vi "..gait set up data vi.vi"() -> ()   [LabVIEW 2018]
uses:
  <vilib>/Analysis/baseanly.llb/Mean (DBL).vi
  <vilib>/University of Leeds/Kinesthesia Toolkit for Microsoft Kinect/_Polymorphic Configure/Event-Skeleton and Video.vi
  <vilib>/University of Leeds/Kinesthesia Toolkit for Microsoft Kinect/_Polymorphic Read/Read-Skeleton and Video.vi
  <vilib>/Utility/file.llb/Write Delimited Spreadsheet (DBL).vi
  <vilib>/University of Leeds/Kinesthesia Toolkit for Microsoft Kinect/_Polymorphic Close/Close-Skeleton and Video.vi
  <vilib>/Utility/file.llb/Read Delimited Spreadsheet (DBL).vi
  <vilib>/Analysis/NI_AALBase.lvlib
panel:
  out "mean calculated":dbl[](array[numeric])
  out "skeleton":refnum<vi>(3d-picture)
  out "?":picture
  out "real time data":dbl[](array[numeric])
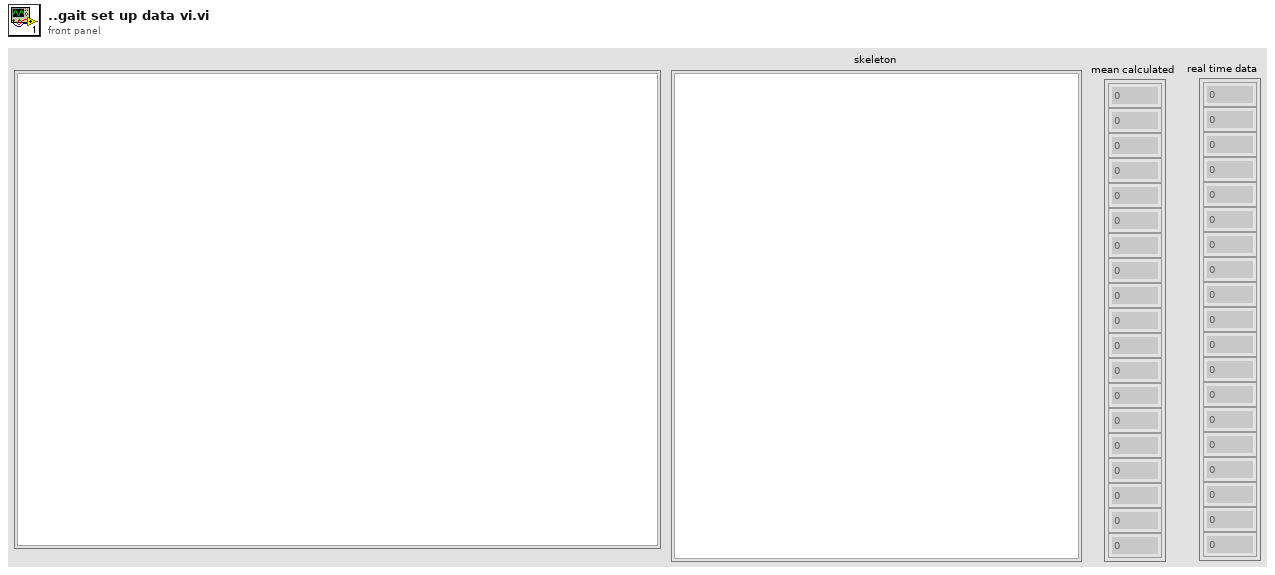
[diagram p1: front panel]
types:
  T1 = enum16{"hip centre", "spine", "shoulder centre", "head", "shoulder left", "elbow left", "wrist left", "hand left", "shoulder right", "elbow right", "wrist right", "hand right", "hip left", "knee left", "ankle left", "foot left", "hip right", "knee right", "ankle right", "foot right"}
  T2 = cluster{cluster{"reference out":refnum<k24>, "KinectSensors":refnum<k24>}, "get_Item":refnum<k24>}
  T3 = cluster{"reference out":refnum<k24>, "KinectSensors":refnum<k24>, "SkeletonStream":refnum<k24>, "ColorStream":refnum<k24>, refnum<k24>[], "get_Item":refnum<k24>}
  T4 = cluster{"Scene":refnum<vi>, "Joints":refnum<vi>[], "Bones":refnum<vi>[]}
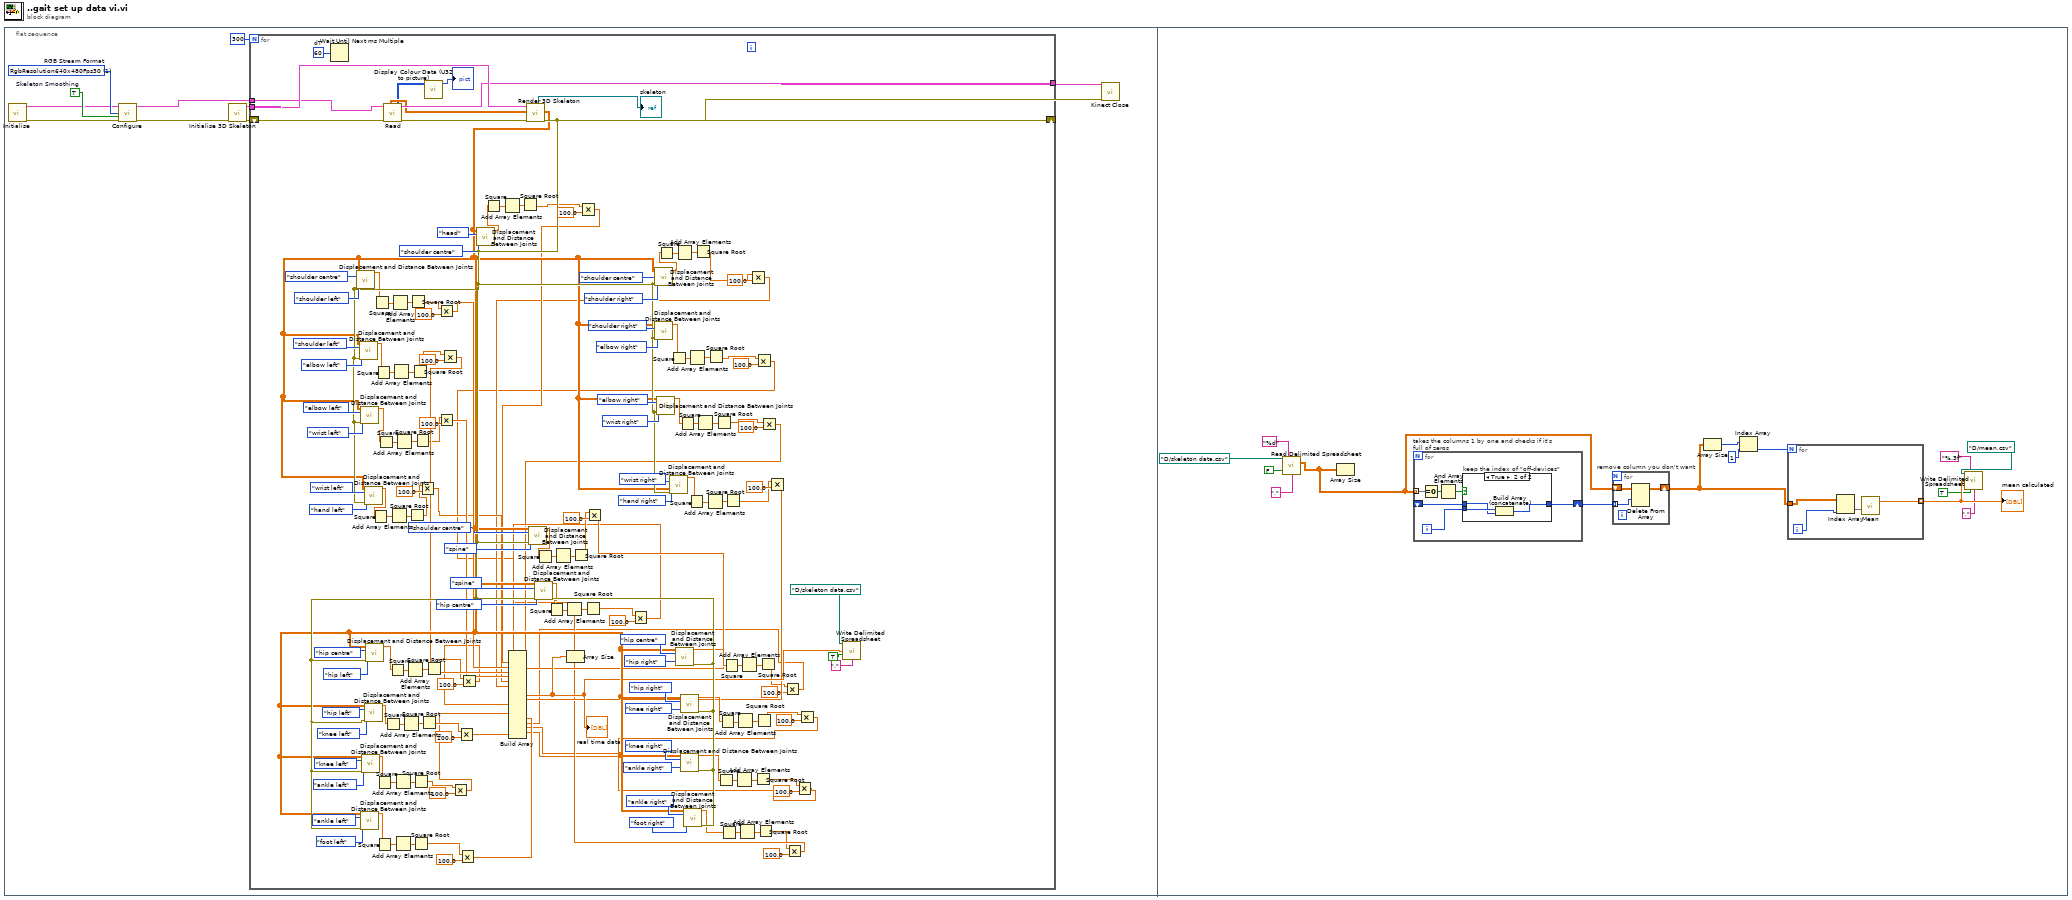
[diagram p0: block diagram]
diagram:
  n1 = flat-sequence {
    frame #0 {
      w7 = 1 items=["Undefined", "RgbResolution640x480Fps30", "RgbResolution1280x960Fps12", "YuvResolution640x480Fps15", "RawYuvResolution640x480Fps15"]  # RGB Stream Format
      w6 = TRUE  # Skeleton Smoothing
      n2 = call <vilib>:"Initialise.vi"() -> ("Kinect References out"=w2:T2, "error out"=w3:errorcluster)  [unwired: 14 in]
      n3 = call-poly <vilib>:"Configure.vi"("Kinect References in"=w2, "RGB Stream Format"=w7, "Skeleton Smoothing"=w6, "error in"=w3) -> ("Kinect References out"=w8:T3, "error out"=w9:errorcluster)  [unwired: 10 in]
      n4 = call <vilib>:"Initialise 3D Skeleton.vi"("error in (no error)"=w9) -> ("error out"=w10:errorcluster, "Scene & Skeleton Refs"=w11:T4)  [unwired: 9 in]
      n5 = for {
        N: 300 -> [_]
        tunnel: [w172] -> w4
        tunnel: w11 -> [w179]
        tunnel: w8 -> [w173]
        shift-right: [w131] -> w5
        shift-left: w10 -> [w175]
        w177 = u32 60  # dT
        n6 = Wait Until Next ms Multiple(millisecond multiple=w177) -> ()  [unwired: 1 out]
        n7 = call-poly <vilib>:"Read.vi"("Kinect References in"=w173, "error in (no error)"=w175) -> ("Primary Skeleton Array"=w171:dbl[][], "Colour output array (U24, RGB)"=w170:u32[][], "Kinect References out"=w172:T3, "error out"=w174:errorcluster)  [unwired: 9 in, 1 out]
        n8 = call <vilib>:"Display Colour Data (U32 to picture).vi"("Colour output array (U24, RGB)"=w170) -> ("new picture"=→"?":picture)  [unwired: 10 in]
        n9 = call <vilib>:"Render 3D Skeleton.vi"("error in (no error)"=w174, "Array of Joint Positions"=w171, "Scene & Skeleton Refs In"=w179) -> ("error out"=w131:errorcluster, "Array of Joint Positions Out"=w130:dbl[][], "Scene Out"=→"skeleton":refnum<vi>)  [unwired: 5 in, 1 out]
        n10 = call <vilib>:"Displacement and Distance Between Joints.vi"("Array of Joint Positions"=w130, "Joint 1"=T1."shoulder centre", "Joint 2"=T1."shoulder left", "error in (no error)"=w131) -> ("X Y Z Displacement Between Joints 1 and 2"=w121:dbl[])  [unwired: 10 in, 1 out]
        n11 = call <vilib>:"Displacement and Distance Between Joints.vi"("Array of Joint Positions"=w130, "Joint 1"=T1."shoulder left", "Joint 2"=T1."elbow left", "error in (no error)"=w131) -> ("X Y Z Displacement Between Joints 1 and 2"=w118:dbl[])  [unwired: 10 in, 1 out]
        n12 = call <vilib>:"Displacement and Distance Between Joints.vi"("Array of Joint Positions"=w130, "Joint 1"=T1."elbow left", "Joint 2"=T1."wrist left", "error in (no error)"=w131) -> ("X Y Z Displacement Between Joints 1 and 2"=w112:dbl[])  [unwired: 10 in, 1 out]
        n13 = call <vilib>:"Displacement and Distance Between Joints.vi"("Array of Joint Positions"=w130, "Joint 1"=T1."ankle left", "Joint 2"=T1."foot left", "error in (no error)"=w131) -> ("X Y Z Displacement Between Joints 1 and 2"=w85:dbl[])  [unwired: 10 in, 1 out]
        n14 = call <vilib>:"Displacement and Distance Between Joints.vi"("Array of Joint Positions"=w130, "Joint 1"=T1."knee left", "Joint 2"=T1."ankle left", "error in (no error)"=w131) -> ("X Y Z Displacement Between Joints 1 and 2"=w86:dbl[])  [unwired: 10 in, 1 out]
        n15 = call <vilib>:"Displacement and Distance Between Joints.vi"("Array of Joint Positions"=w130, "Joint 1"=T1."wrist left", "Joint 2"=T1."hand left", "error in (no error)"=w131) -> ("X Y Z Displacement Between Joints 1 and 2"=w102:dbl[])  [unwired: 10 in, 1 out]
        n16 = call <vilib>:"Displacement and Distance Between Joints.vi"("Array of Joint Positions"=w130, "Joint 1"=T1."hip left", "Joint 2"=T1."knee left", "error in (no error)"=w131) -> ("X Y Z Displacement Between Joints 1 and 2"=w87:dbl[])  [unwired: 10 in, 1 out]
        n17 = call <vilib>:"Displacement and Distance Between Joints.vi"("Array of Joint Positions"=w130, "Joint 1"=T1."hip centre", "Joint 2"=T1."hip left", "error in (no error)"=w131) -> ("X Y Z Displacement Between Joints 1 and 2"=w94:dbl[])  [unwired: 10 in, 1 out]
        n18 = Square(x=w102) -> (x^2=w106:dbl[])
        n19 = Square(x=w121) -> (x^2=w123:dbl[])
        n20 = Square(x=w118) -> (x^2=w120:dbl[])
        n21 = Square(x=w86) -> (x^2=w91:dbl[])
        n22 = Square(x=w85) -> (x^2=w89:dbl[])
        n23 = Square(x=w112) -> (x^2=w114:dbl[])
        n24 = Square(x=w87) -> (x^2=w93:dbl[])
        n25 = Square(x=w94) -> (x^2=w96:dbl[])
        n26 = Add Array Elements(numeric array=w106) -> (sum=w105:dbl)
        n27 = Add Array Elements(numeric array=w123) -> (sum=w122:dbl)
        n28 = Add Array Elements(numeric array=w120) -> (sum=w119:dbl)
        n29 = Add Array Elements(numeric array=w91) -> (sum=w90:dbl)
        n30 = Add Array Elements(numeric array=w89) -> (sum=w88:dbl)
        n31 = Add Array Elements(numeric array=w114) -> (sum=w113:dbl)
        n32 = Add Array Elements(numeric array=w93) -> (sum=w92:dbl)
        n33 = Add Array Elements(numeric array=w96) -> (sum=w95:dbl)
        n34 = Square Root(x=w105) -> (sqrt(x)=w55:dbl)
        n35 = Square Root(x=w122) -> (sqrt(x)=w63:dbl)
        n36 = Square Root(x=w119) -> (sqrt(x)=w60:dbl)
        n37 = Square Root(x=w90) -> (sqrt(x)=w28:dbl)
        n38 = Square Root(x=w88) -> (sqrt(x)=w25:dbl)
        n39 = Square Root(x=w113) -> (sqrt(x)=w57:dbl)
        n40 = Multiply(x=w55, y=100.0) -> (x*y=w54:dbl)
        n41 = Square Root(x=w92) -> (sqrt(x)=w31:dbl)
        n42 = Square Root(x=w95) -> (sqrt(x)=w34:dbl)
        n43 = Multiply(x=w63, y=100.0) -> (x*y=w64:dbl)
        n44 = Multiply(x=w57, y=100.0) -> (x*y=w58:dbl)
        n45 = Multiply(x=w60, y=100.0) -> (x*y=w61:dbl)
        n46 = Multiply(x=w28, y=100.0) -> (x*y=w27:dbl)
        n47 = Multiply(x=w31, y=100.0) -> (x*y=w30:dbl)
        n48 = Multiply(x=w25, y=100.0) -> (x*y=w24:dbl)
        n49 = Multiply(x=w34, y=100.0) -> (x*y=w33:dbl)
        n50 = call <vilib>:"Displacement and Distance Between Joints.vi"("Array of Joint Positions"=w130, "Joint 1"=T1."head", "Joint 2"=T1."shoulder centre", "error in (no error)"=w131) -> ("X Y Z Displacement Between Joints 1 and 2"=w127:dbl[])  [unwired: 10 in, 1 out]
        n51 = Square(x=w127) -> (x^2=w129:dbl[])
        n52 = Add Array Elements(numeric array=w129) -> (sum=w128:dbl)
        n53 = Square Root(x=w128) -> (sqrt(x)=w66:dbl)
        n54 = call <vilib>:"Displacement and Distance Between Joints.vi"("Array of Joint Positions"=w130, "Joint 1"=T1."shoulder centre", "Joint 2"=T1."spine", "error in (no error)"=w131) -> ("X Y Z Displacement Between Joints 1 and 2"=w100:dbl[])  [unwired: 10 in, 1 out]
        n55 = call <vilib>:"Displacement and Distance Between Joints.vi"("Array of Joint Positions"=w130, "Joint 1"=T1."spine", "Joint 2"=T1."hip centre", "error in (no error)"=w131) -> ("X Y Z Displacement Between Joints 1 and 2"=w97:dbl[])  [unwired: 10 in, 1 out]
        n56 = Square(x=w100) -> (x^2=w108:dbl[])
        n57 = Square(x=w97) -> (x^2=w99:dbl[])
        n58 = Add Array Elements(numeric array=w108) -> (sum=w107:dbl)
        n59 = Add Array Elements(numeric array=w99) -> (sum=w98:dbl)
        n60 = Square Root(x=w107) -> (sqrt(x)=w52:dbl)
        n61 = Multiply(x=w66, y=100.0) -> (x*y=w67:dbl)
        n62 = Square Root(x=w98) -> (sqrt(x)=w48:dbl)
        n63 = Multiply(x=w52, y=100.0) -> (x*y=w51:dbl)
        n64 = Multiply(x=w48, y=100.0) -> (x*y=w49:dbl)
        n65 = call <vilib>:"Displacement and Distance Between Joints.vi"("Array of Joint Positions"=w130, "Joint 1"=T1."shoulder centre", "Joint 2"=T1."shoulder right", "error in (no error)"=w131) -> ("X Y Z Displacement Between Joints 1 and 2"=w124:dbl[])  [unwired: 10 in, 1 out]
        n66 = call <vilib>:"Displacement and Distance Between Joints.vi"("Array of Joint Positions"=w130, "Joint 1"=T1."shoulder right", "Joint 2"=T1."elbow right", "error in (no error)"=w131) -> ("X Y Z Displacement Between Joints 1 and 2"=w115:dbl[])  [unwired: 10 in, 1 out]
        n67 = call <vilib>:"Displacement and Distance Between Joints.vi"("Array of Joint Positions"=w130, "Joint 1"=T1."elbow right", "Joint 2"=T1."wrist right", "error in (no error)"=w131) -> ("X Y Z Displacement Between Joints 1 and 2"=w109:dbl[])  [unwired: 10 in, 1 out]
        n68 = Square(x=w124) -> (x^2=w126:dbl[])
        n69 = call <vilib>:"Displacement and Distance Between Joints.vi"("Array of Joint Positions"=w130, "Joint 1"=T1."wrist right", "Joint 2"=T1."hand right", "error in (no error)"=w131) -> ("X Y Z Displacement Between Joints 1 and 2"=w101:dbl[])  [unwired: 10 in, 1 out]
        n70 = Square(x=w115) -> (x^2=w117:dbl[])
        n71 = Add Array Elements(numeric array=w126) -> (sum=w125:dbl)
        n72 = call <vilib>:"Displacement and Distance Between Joints.vi"("Array of Joint Positions"=w130, "Joint 1"=T1."hip centre", "Joint 2"=T1."hip right", "error in (no error)"=w131) -> ("X Y Z Displacement Between Joints 1 and 2"=w82:dbl[])  [unwired: 10 in, 1 out]
        n73 = Square(x=w109) -> (x^2=w111:dbl[])
        n74 = call <vilib>:"Displacement and Distance Between Joints.vi"("Array of Joint Positions"=w130, "Joint 1"=T1."hip right", "Joint 2"=T1."knee right", "error in (no error)"=w131) -> ("X Y Z Displacement Between Joints 1 and 2"=w75:dbl[])  [unwired: 10 in, 1 out]
        n75 = call <vilib>:"Displacement and Distance Between Joints.vi"("Array of Joint Positions"=w130, "Joint 1"=T1."knee right", "Joint 2"=T1."ankle right", "error in (no error)"=w131) -> ("X Y Z Displacement Between Joints 1 and 2"=w74:dbl[])  [unwired: 10 in, 1 out]
        n76 = call <vilib>:"Displacement and Distance Between Joints.vi"("Array of Joint Positions"=w130, "Joint 1"=T1."ankle right", "Joint 2"=T1."foot right", "error in (no error)"=w131) -> ("X Y Z Displacement Between Joints 1 and 2"=w73:dbl[])  [unwired: 10 in, 1 out]
        n77 = Square(x=w101) -> (x^2=w104:dbl[])
        n78 = Add Array Elements(numeric array=w117) -> (sum=w116:dbl)
        n79 = Square Root(x=w125) -> (sqrt(x)=w46:dbl)
        n80 = Add Array Elements(numeric array=w111) -> (sum=w110:dbl)
        n81 = Add Array Elements(numeric array=w104) -> (sum=w103:dbl)
        n82 = Square Root(x=w116) -> (sqrt(x)=w42:dbl)
        n83 = Square Root(x=w110) -> (sqrt(x)=w40:dbl)
        n84 = Square(x=w74) -> (x^2=w79:dbl[])
        n85 = Square(x=w75) -> (x^2=w81:dbl[])
        n86 = Square(x=w73) -> (x^2=w76:dbl[])
        n87 = Square(x=w82) -> (x^2=w84:dbl[])
        n88 = Square Root(x=w103) -> (sqrt(x)=w37:dbl)
        n89 = Add Array Elements(numeric array=w79) -> (sum=w78:dbl)
        n90 = Add Array Elements(numeric array=w81) -> (sum=w80:dbl)
        n91 = Add Array Elements(numeric array=w76) -> (sum=w77:dbl)
        n92 = Add Array Elements(numeric array=w84) -> (sum=w83:dbl)
        n93 = Multiply(x=w46, y=100.0) -> (x*y=w45:dbl)
        n94 = Square Root(x=w78) -> (sqrt(x)=w18:dbl)
        n95 = Multiply(x=w42, y=100.0) -> (x*y=w43:dbl)
        n96 = Square Root(x=w80) -> (sqrt(x)=w16:dbl)
        n97 = Square Root(x=w77) -> (sqrt(x)=w21:dbl)
        n98 = Square Root(x=w83) -> (sqrt(x)=w13:dbl)
        n99 = Multiply(x=w40, y=100.0) -> (x*y=w39:dbl)
        n100 = Multiply(x=w37, y=100.0) -> (x*y=w36:dbl)
        n101 = Multiply(x=w13, y=100.0) -> (x*y=w12:dbl)
        n102 = Multiply(x=w21, y=100.0) -> (x*y=w22:dbl)
        n103 = Multiply(x=w18, y=100.0) -> (x*y=w19:dbl)
        n104 = Multiply(x=w16, y=100.0) -> (x*y=w15:dbl)
        n105 = Build Array(w49, w51, w67, w64, w61, w58, w54, w45, w43, w39, w36, w33, w30, w27, w24, w12, w15, w19, w22) -> (w69:dbl[])
        "real time data" <- w69
        n106 = Array Size(array=w69) -> ()  [unwired: 1 out]
        n107 = call-poly <vilib>:"Write Delimited Spreadsheet.vi"("file path (dialog if empty)"=path "D:/skeleton data.csv", "1D data"=w69, "append to file? (new file:F)"=TRUE, "delimiter (\\t)"="," ("delimiter (\\t)")) -> ()  [unwired: 10 in, 2 out]
      }
      n108 = call-poly <vilib>:"Kinect Close.vi"("Kinect References in"=w4, "error in"=w5) -> ()  [unwired: 13 in, 1 out]
    }
    frame #1 {
      n109 = call-poly <vilib>:"Read Delimited Spreadsheet.vi"("file path (dialog if empty)"=path "D:/skeleton data.csv" ("file path (dialog if empty) 2"), "format (%.3f)"="%d", "transpose? (F)"=FALSE, "delimiter (\\t)"="," ("delimiter (\\t)")) -> ("all rows"=w191:dbl[][])  [unwired: 6 in, 5 out]
      n110 = Array Size(array=w191) -> ()  [unwired: 1 out]
      n111 = for "takes the columns 1 by one and checks if it's full of zeros" {
        tunnel: w191 -> [w203] mode=indexing
        shift-right: [w201] -> w192
        shift-left: _ -> [w202]
        i -> [w200]
        n112 = Equal To 0?(x=w203) -> (x = 0?=w199:bool[])
        n113 = And Array Elements(Boolean array=w199) -> (logical AND=w198:bool)
        n114 = case "keep the index of \"off-devices\"" shown="True" w198 {
          tunnel: w202 -> [w204 w205]
          tunnel: [w204 w207] -> w201
          tunnel: w200 -> [_ w206]
          frame False {
          }
          frame True {
            n115 = Build Array (concatenate)(w206, w205) -> (w207:i32[])
          }
        }
      }
      n116 = for "remove column you don't want" {
        shift-right: [w196] -> w187
        shift-left: w191 -> [w197]
        tunnel: w192 -> [w195] mode=indexing
        n117 = Delete From Array(array=w197, index (row)=w195) -> (array with subset deleted=w196:dbl[][])  [unwired: 2 in, 1 out]
      }
      n118 = Array Size(array=w187) -> (size(s)=w189:i32[])
      n119 = Index Array(array=w189, index=1) -> (element=w188:i32)
      n120 = for {
        N: w188 -> [_]
        tunnel: w187 -> [w211]
        tunnel: [w208] -> w185 mode=indexing
        i -> [w210]
        n121 = Index Array(array=w211, index (col)=w210) -> (element=w209:dbl[])  [unwired: 1 in]
        n122 = call-poly <vilib>:"Mean.vi"("X"=w209) -> ("mean"=w208:dbl)  [unwired: 1 out]
      }
      "mean calculated" <- w185
      n123 = call-poly <vilib>:"Write Delimited Spreadsheet.vi"("file path (dialog if empty)"=path "D:/mean.csv" ("file path (dialog if empty) 3"), "format (%.3f)"="%.3f", "1D data"=w185, "transpose? (no:F)"=TRUE, "delimiter (\\t)"="," ("delimiter (\\t)")) -> ()  [unwired: 9 in, 2 out]
    }
  }
